vi "DisposeCore.vi"(8 "error in (no error)":errorcluster, 11 "CreatorB":refnum<class "CreatorB.lvclass">) -> (0 "error out":errorcluster, 3 "CreatorB":refnum<class "CreatorB.lvclass">)   [LabVIEW 2020, in "FactoryMethod.lvlib" / "FactoryMethodLazyEvaluation.lvlib" / "CreatorB.lvclass"]
uses:
  CreatorB.lvclass
  Private/TypeDef/privateDataDVR.ctl
  Private/TypeDef/privateData.ctl
  CreatorB.lvclass/CreatorB.ctl
  Creator/Creator.lvclass
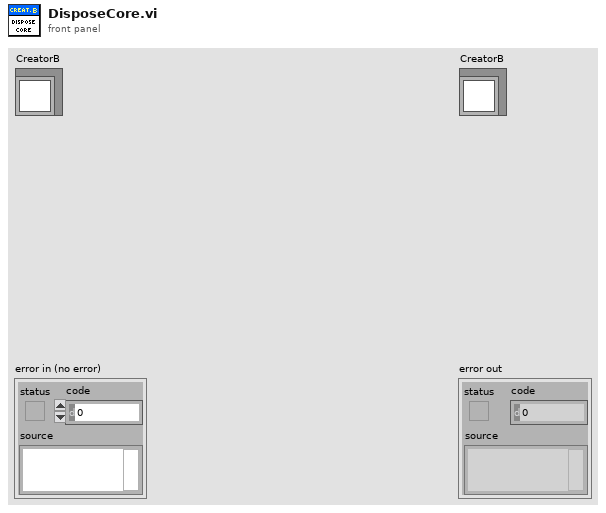
[diagram p1: front panel]
types:
  T1 = typedef "FactoryMethod.lvlib/FactoryMethodLazyEvaluation.lvlib/CreatorB.lvclass/privateDataDVR.ctl" = refnum<data-value>
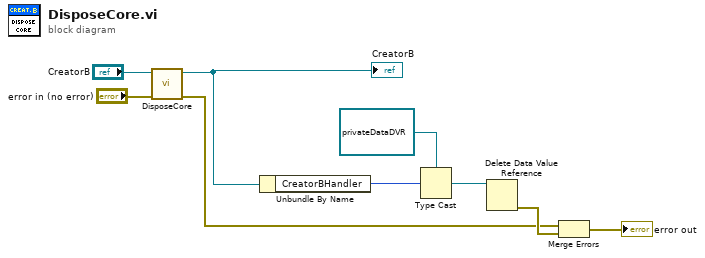
[diagram p0: block diagram]
diagram:
  n1 = call-parent "DisposeCore.vi"("error in (no error)"="error in (no error)", "Creator in"="CreatorB") -> ("error out"=w2:errorcluster, "Creator out"=w1:refnum<class "CreatorB.lvclass">)  [unwired: 8 in]
  "CreatorB" <- w1
  n2 = Unbundle By Name(w1) -> ("CreatorBHandler"=w6:u32)
  n3 = Type Cast(type=T1 refnum ("privateDataDVR"), x=w6) -> (*(type *) &x=w7:T1)
  n4 = Delete Data Value Reference(data value reference=w7) -> (error out=w4:errorcluster)  [unwired: 1 in, 1 out]
  n5 = Merge Errors(w2, w4) -> (→"error out":errorcluster)
